vi "Pfeiffer-RVC300.ProcCases.vi"(0 "i ref in":refnum<vi>, 1 "selector":string, 2 "Data":T1, 3 "call cluster":T2={"Object"="", "Selector"="", "CallType"=enum."synchronous", "Async Object"="", "Async Selector"="", "Data Descriptor"="", "Data"=[], "Error #"=0, "Expire"=0}, 5 "error in (no error)":errorcluster) -> (14 "i ref out":refnum<vi>, 17 "answer cluster":T2={"Object"="", "Selector"="", "CallType"=enum."synchronous", "Async Object"="", "Async Selector"="", "Data Descriptor"="", "Data"=[], "Error #"=0, "Expire"=0}, 19 "error out":errorcluster)   [LabVIEW 2014, in "Pfeiffer-RVC300.lvlib"]
doc: "This method is called by a process from within the default case in the event loop. The methods of a class that are linked to events will be called from THIS method. Add your code here."
uses:
  Pfeiffer-RVC300.lvlib
  CS_Core/CSSystem/CoreLib/CoreLib.lvlib
  CS_Core/BaseProcess/BaseProcess.lvlib
  CS_Core/CSApplicationBaseClasses/DeviceBase/DeviceBase.lvlib
  CS_Core/CSSystem/CoreLib/CoreLib.string 2 byte array.vi
  CS_Core/CSSystem/CoreLib/CoreLib.byte array 2 double.vi
  CS_Core/CSSystem/CoreLib/CoreLib.double 2 byte array.vi
  CS_Core/CSSystem/CoreLib/CoreLib.byte array 2 short.vi
  CS_Core/CSSystem/CoreLib/CoreLib.int 2 byte array.vi
  CS_Core/CSSystem/CoreLib/CoreLib.byte array 2 int.vi
  CS_Core/CSSystem/CoreDefs/CoreDefs.call_type.ctl
  CS_Core/CSSystem/CoreDefs/CoreDefs.rawDataType.ctl
  CS_Core/BaseProcess/BaseProcess.descriptor string definition.ctl
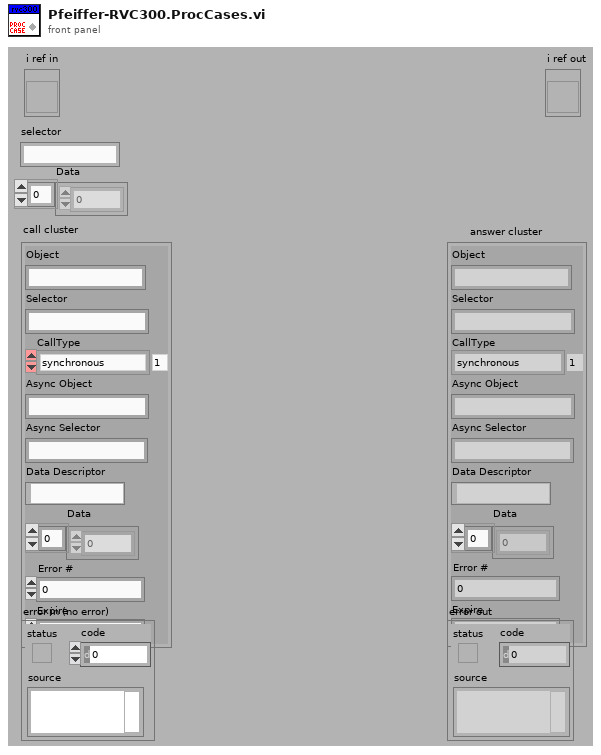
[diagram p1: front panel]
types:
  T1 = typedef "CoreDefs.rawDataType.ctl" = i8[]
  T2 = typedef "CoreDefs.call_type.ctl" = cluster{"Object":string, "Selector":string, "CallType":enum16{"simple", "synchronous", "asynchronous"}, "Async Object":string, "Async Selector":string, "Data Descriptor":T3, "Data":T1, "Error #":i32, "Expire":u32}
  T3 = typedef "BaseProcess.lvlib/BaseProcess.descriptor string definition.ctl" = string
  T4 = typedef "Pfeiffer-RVC300.lvlib/Pfeiffer-RVC300.regulation mode.ctl" = enum16{"unknown", "Pressure", "Flow", "Wait"}
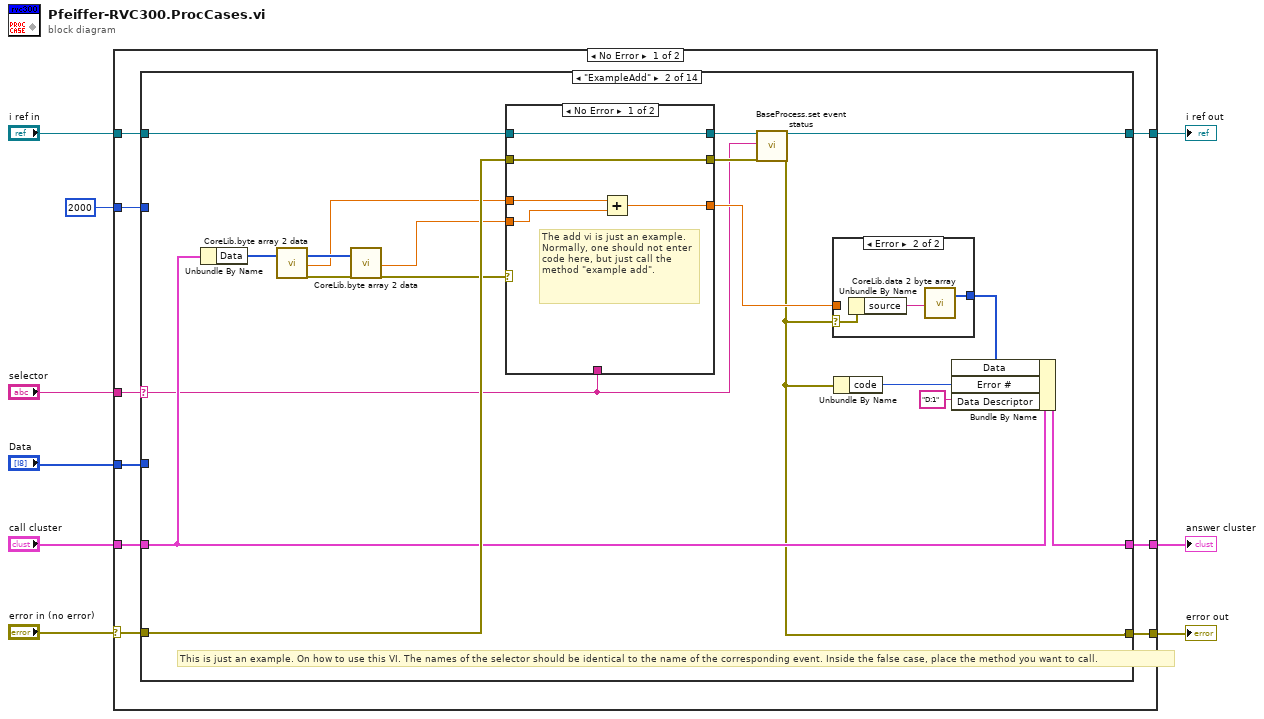
[diagram p0: block diagram]
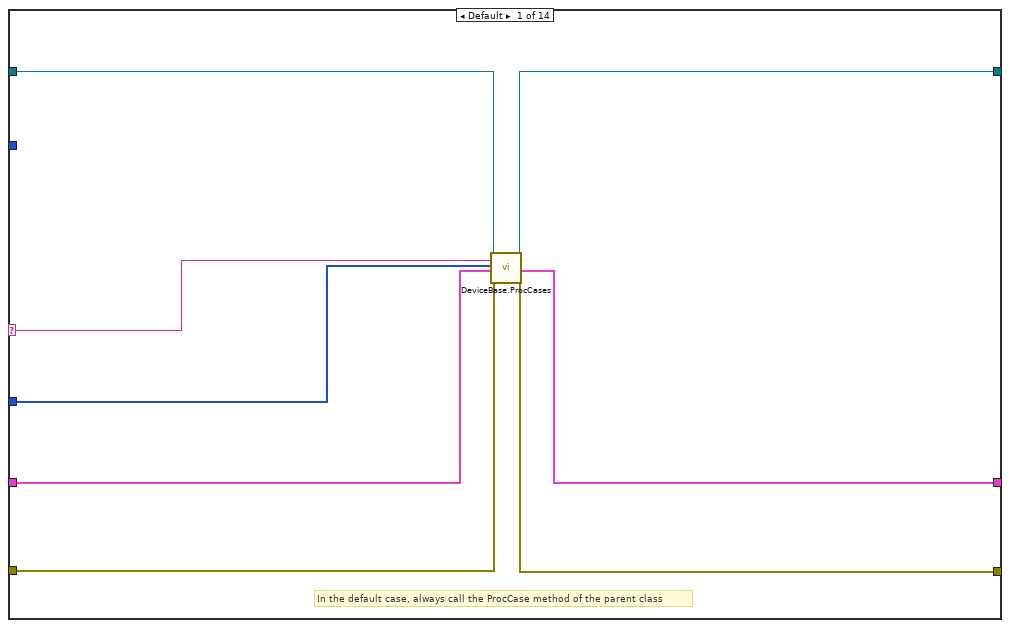
[diagram p2: hidden frame]
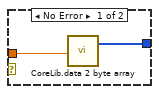
[diagram p3: hidden frame]
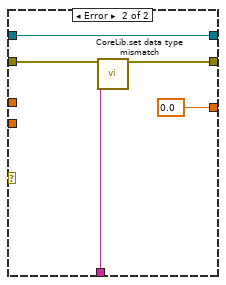
[diagram p4: hidden frame]
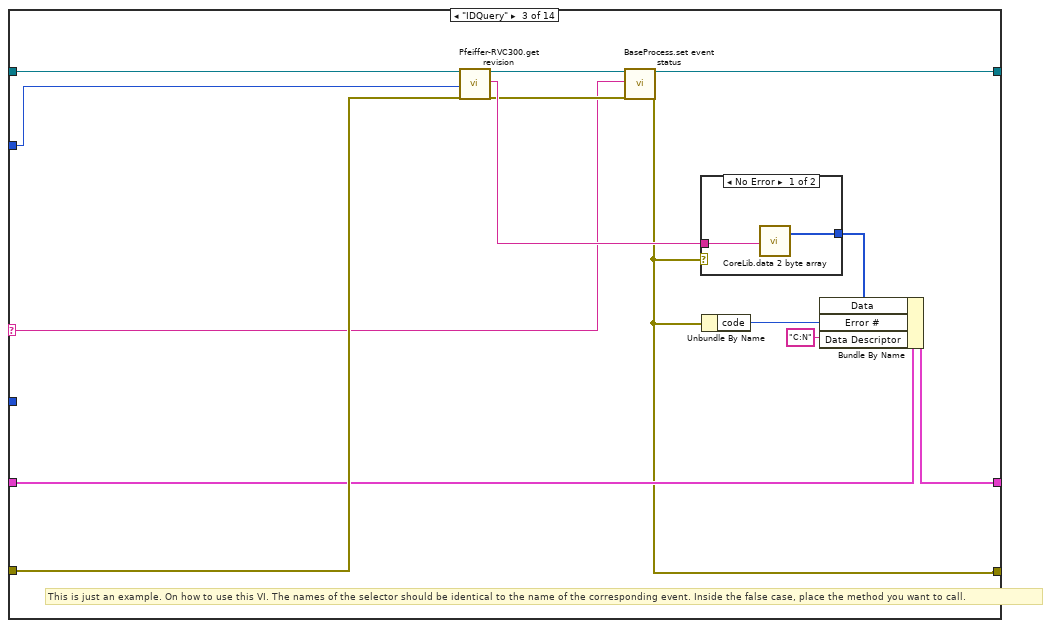
[diagram p5: hidden frame]
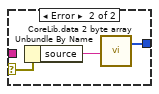
[diagram p6: hidden frame]
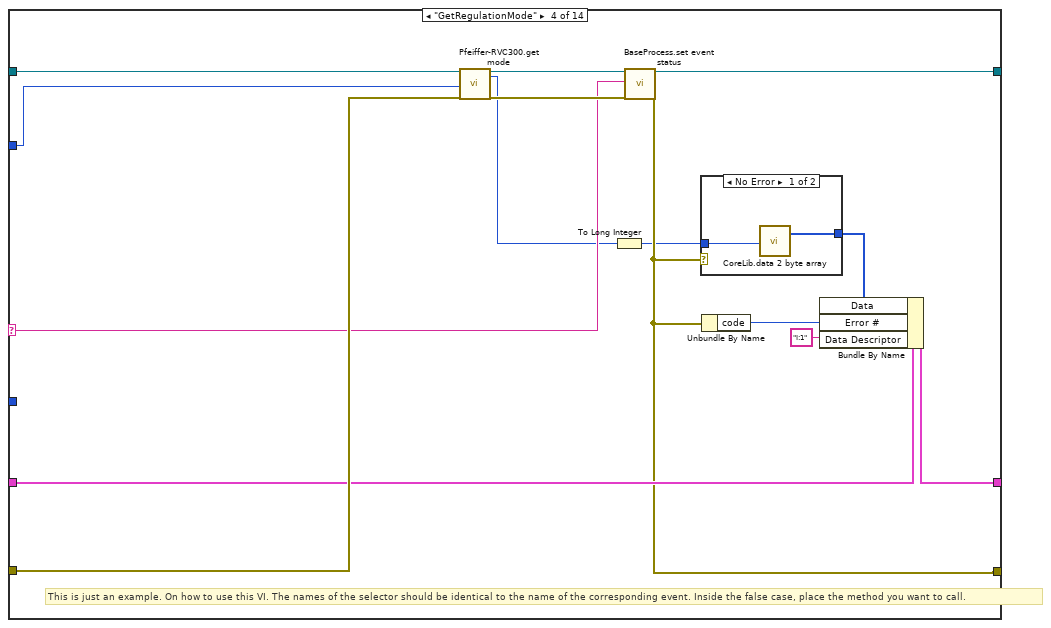
[diagram p7: hidden frame]
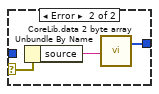
[diagram p8: hidden frame]
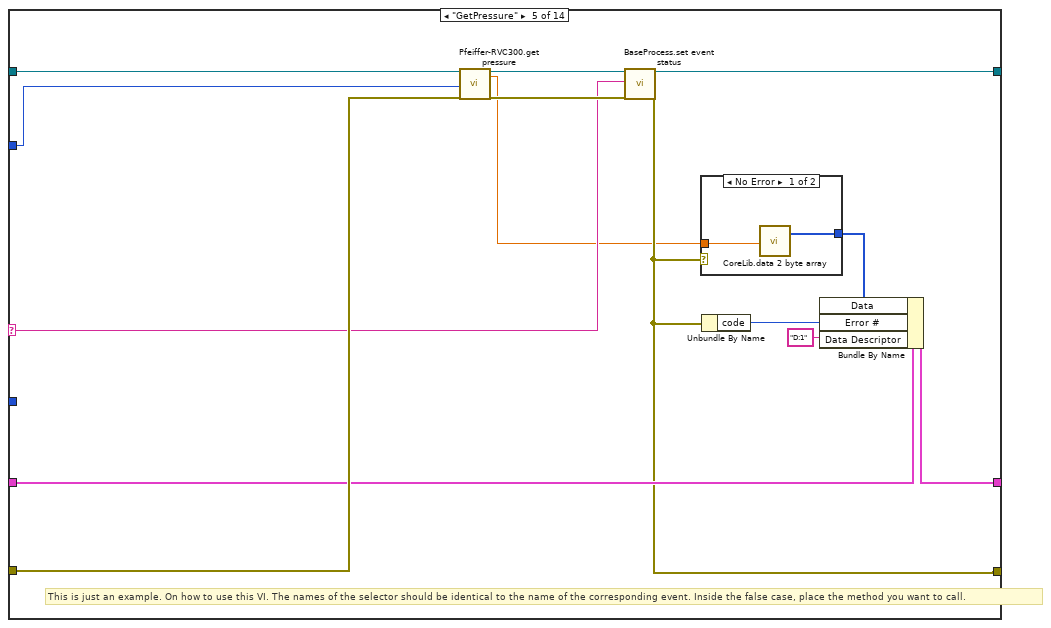
[diagram p9: hidden frame]
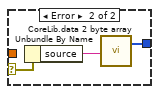
[diagram p10: hidden frame]
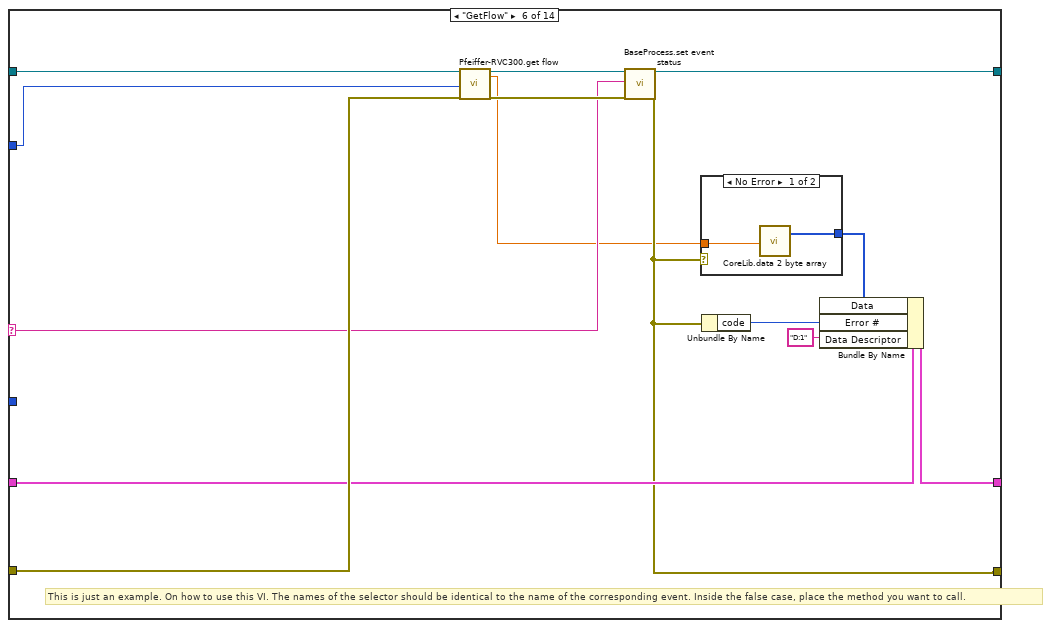
[diagram p11: hidden frame]
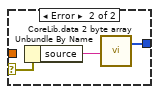
[diagram p12: hidden frame]
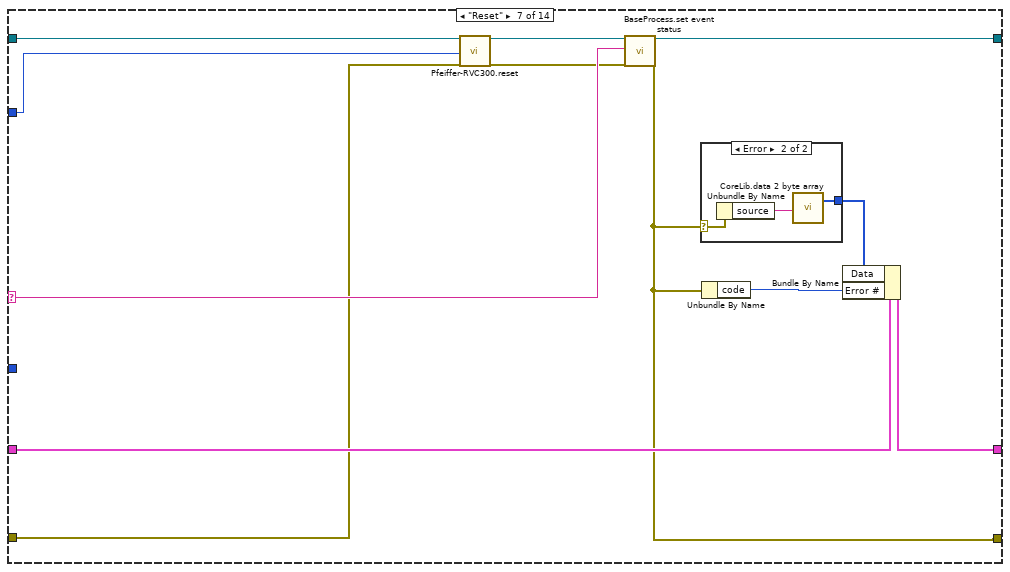
[diagram p13: hidden frame]
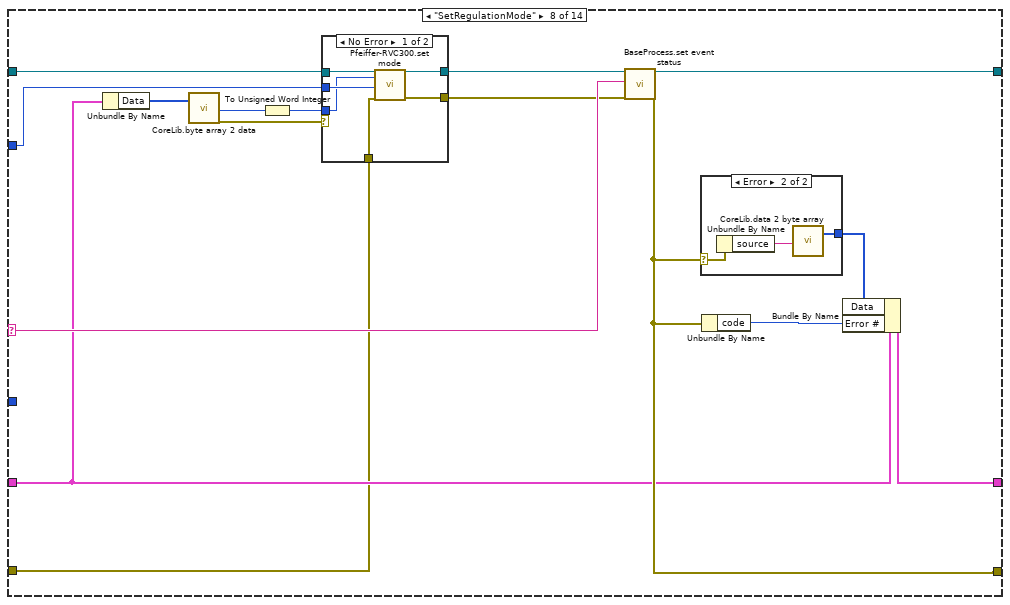
[diagram p15: hidden frame]
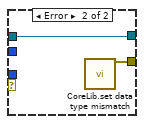
[diagram p16: hidden frame]
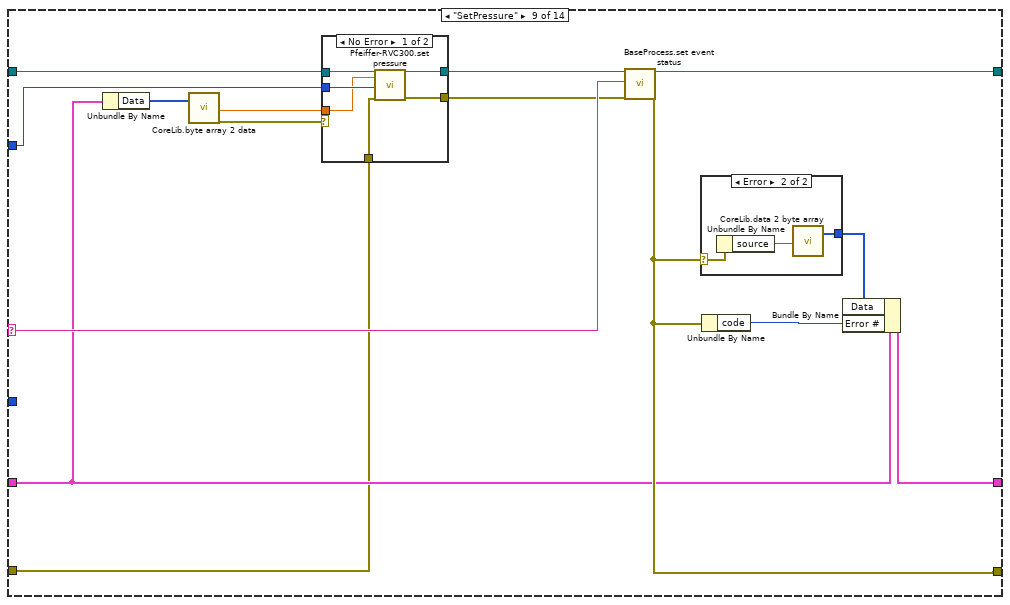
[diagram p18: hidden frame]
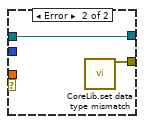
[diagram p19: hidden frame]
diagram:
  n1 = case shown="No Error" "error in (no error)" {
    selector: "error in (no error)" -> [w11 w314]
    tunnel: "selector" -> [w18 _]
    tunnel: [w17 w315] -> w8
    tunnel: "Data" -> [w16 _]
    tunnel: "call cluster" -> [w15 w315]
    tunnel: "i ref in" -> [w14 w316]
    tunnel: [w13 w316] -> w4
    tunnel: [w12 w314] -> w3
    tunnel: 2000 -> [w10 _]
    frame No Error {
      n2 = case shown="\"ExampleAdd\"" w18 {
        selector: w18 -> [w21 w35 w64 w85 w104 w123 w144 w163 w188 w213 w235 w250 w268 w301]
        tunnel: w16 -> [w19 _ _ _ _ _ _ _ _ _ _ _ _ _]
        tunnel: w14 -> [w20 w45 w74 w94 w113 w132 w142 w158 w183 w208 w233 w248 w278 w310]
        tunnel: [w26 w34 w63 w84 w103 w122 w143 w162 w187 w212 w234 w249 w267 w300] -> w13
        tunnel: w15 -> [w22 w41 w70 w91 w110 w129 w148 w159 w184 w209 w239 w254 w274 w307]
        tunnel: [w23 w40 w69 w90 w109 w128 w147 w166 w191 w216 w238 w253 w273 w306] -> w17
        tunnel: w11 -> [w25 w44 w73 w93 w112 w131 w139 w156 w181 w206 w230 w245 w277 w309]
        tunnel: [w24 w36 w65 w86 w105 w124 w145 w164 w189 w214 w236 w251 w269 w302] -> w12
        tunnel: w10 -> [_ _ w61 w82 w101 w120 w138 w154 w180 w205 w229 w244 w259 w299]
        frame Default {
          # "In the default case, always call the ProcCase method of the parent class"
          n3 = call "DeviceBase.ProcCases.vi"("i ref in"=w20, "selector"=w21, "Data"=w19, "call cluster"=w22, "error in (no error)"=w25) -> ("i ref out"=w26:refnum<vi>, "answer cluster"=w23:T2, "error out"=w24:errorcluster)  [unwired: 12 in]
        }
        frame "ExampleAdd" {
          # "This is just an example. On how to use this VI. The names of the selector should be identical to the name of the corresponding event. Inside the false case, place the method you want to call."
          n4 = Unbundle By Name(w41) -> ("Data"=w32:T1)
          n5 = call-poly "CoreLib.byte array 2 data.vi"("byteArray"=w32) -> ("byteArray out"=w30:T1, "d64"=w28:dbl, "error out"=w31:errorcluster)  [unwired: 16 in]
          n6 = call-poly "CoreLib.byte array 2 data.vi"("byteArray"=w30, "error in (no error)"=w31) -> ("d64"=w27:dbl, "error out"=w29:errorcluster)  [unwired: 15 in, 1 out]
          n7 = case shown="No Error" w29 {
            tunnel: [w52 w60] -> w38
            tunnel: w45 -> [w52 w60]
            tunnel: w44 -> [w53 w59]
            tunnel: [w53 w58] -> w37
            tunnel: w27 -> [w55 _]
            tunnel: [w54 0.0] -> w43
            tunnel: w35 -> [_ w56]
            tunnel: w28 -> [w51 _]
            frame No Error {
              # "The add vi is just an example. Normally, one should not enter code here, but just call the method \"example add\"."
              n8 = Add(x=w51, y=w55) -> (x+y=w54:dbl)
            }
            frame Error {
              n9 = call "CoreLib.set data type mismatch.vi"("error in (no error)"=w59, "error source"=w56) -> ("error out"=w58:errorcluster)  [unwired: 17 in]
            }
          }
          n10 = call "BaseProcess.set event status.vi"("i ref in"=w38, "EventStatus"=w35, "error in (no error)"=w37) -> ("i ref out"=w34:refnum<vi>, "error out"=w36:errorcluster)  [unwired: 14 in, 1 out]
          n11 = case shown="Error" w36 {
            selector: w36 -> [_ w50]
            tunnel: [w46 w49] -> w39
            tunnel: w43 -> [w47 _]
            frame No Error {
              n12 = call-poly "CoreLib.data 2 byte array.vi"("f64"=w47) -> ("byteArray out"=w46:T1)  [unwired: 18 in]
            }
            frame Error {
              n13 = Unbundle By Name(w50) -> ("source"=w48:string)
              n14 = call-poly "CoreLib.data 2 byte array.vi"("string"=w48) -> ("byteArray out"=w49:T1)  [unwired: 18 in]
            }
          }
          n15 = Unbundle By Name(w36) -> ("code"=w42:i32)
          n16 = Bundle By Name(cluster=w41, "Data"=w39, "Error #"=w42, "Data Descriptor"="D:1") -> (w40:T2)
        }
        frame "IDQuery" {
          # "This is just an example. On how to use this VI. The names of the selector should be identical to the name of the corresponding event. Inside the false case, place the method you want to call."
          n17 = call "Pfeiffer-RVC300.get revision.vi"("i ref in"=w74, "ms timeout (10000)"=w61, "error in (no error)"=w73) -> ("i ref out"=w67:refnum<vi>, "revision"=w72:string, "error out"=w66:errorcluster)  [unwired: 13 in, 1 out]
          n18 = call "BaseProcess.set event status.vi"("i ref in"=w67, "EventStatus"=w64, "error in (no error)"=w66) -> ("i ref out"=w63:refnum<vi>, "error out"=w65:errorcluster)  [unwired: 14 in, 1 out]
          n19 = case shown="No Error" w65 {
            selector: w65 -> [_ w79]
            tunnel: [w76 w78] -> w68
            tunnel: w72 -> [w75 _]
            frame No Error {
              n20 = call-poly "CoreLib.data 2 byte array.vi"("string"=w75) -> ("byteArray out"=w76:T1)  [unwired: 18 in]
            }
            frame Error {
              n21 = Unbundle By Name(w79) -> ("source"=w77:string)
              n22 = call-poly "CoreLib.data 2 byte array.vi"("string"=w77) -> ("byteArray out"=w78:T1)  [unwired: 18 in]
            }
          }
          n23 = Unbundle By Name(w65) -> ("code"=w71:i32)
          n24 = Bundle By Name(cluster=w70, "Data"=w68, "Error #"=w71, "Data Descriptor"="C:N") -> (w69:T2)
        }
        frame "GetRegulationMode" {
          # "This is just an example. On how to use this VI. The names of the selector should be identical to the name of the corresponding event. Inside the false case, place the method you want to call."
          n25 = call "Pfeiffer-RVC300.get mode.vi"("i ref in"=w94, "ms timeout (10000)"=w82, "error in (no error)"=w93) -> ("i ref out"=w88:refnum<vi>, "regulationMode"=w81:T4, "error out"=w87:errorcluster)  [unwired: 13 in, 1 out]
          n26 = To Long Integer(number=w81) -> (32bit integer=w80:i32)
          n27 = call "BaseProcess.set event status.vi"("i ref in"=w88, "EventStatus"=w85, "error in (no error)"=w87) -> ("i ref out"=w84:refnum<vi>, "error out"=w86:errorcluster)  [unwired: 14 in, 1 out]
          n28 = case shown="No Error" w86 {
            selector: w86 -> [_ w99]
            tunnel: [w96 w98] -> w89
            tunnel: w80 -> [w95 _]
            frame No Error {
              n29 = call-poly "CoreLib.data 2 byte array.vi"("i32"=w95) -> ("byteArray out"=w96:T1)  [unwired: 18 in]
            }
            frame Error {
              n30 = Unbundle By Name(w99) -> ("source"=w97:string)
              n31 = call-poly "CoreLib.data 2 byte array.vi"("string"=w97) -> ("byteArray out"=w98:T1)  [unwired: 18 in]
            }
          }
          n32 = Unbundle By Name(w86) -> ("code"=w92:i32)
          n33 = Bundle By Name(cluster=w91, "Data"=w89, "Error #"=w92, "Data Descriptor"="I:1") -> (w90:T2)
        }
        frame "GetPressure" {
          # "This is just an example. On how to use this VI. The names of the selector should be identical to the name of the corresponding event. Inside the false case, place the method you want to call."
          n34 = call "Pfeiffer-RVC300.get pressure.vi"("i ref in"=w113, "ms timeout (10000)"=w101, "error in (no error)"=w112) -> ("i ref out"=w107:refnum<vi>, "pressure"=w100:dbl, "error out"=w106:errorcluster)  [unwired: 13 in, 1 out]
          n35 = call "BaseProcess.set event status.vi"("i ref in"=w107, "EventStatus"=w104, "error in (no error)"=w106) -> ("i ref out"=w103:refnum<vi>, "error out"=w105:errorcluster)  [unwired: 14 in, 1 out]
          n36 = case shown="No Error" w105 {
            selector: w105 -> [_ w118]
            tunnel: [w115 w117] -> w108
            tunnel: w100 -> [w114 _]
            frame No Error {
              n37 = call-poly "CoreLib.data 2 byte array.vi"("f64"=w114) -> ("byteArray out"=w115:T1)  [unwired: 18 in]
            }
            frame Error {
              n38 = Unbundle By Name(w118) -> ("source"=w116:string)
              n39 = call-poly "CoreLib.data 2 byte array.vi"("string"=w116) -> ("byteArray out"=w117:T1)  [unwired: 18 in]
            }
          }
          n40 = Unbundle By Name(w105) -> ("code"=w111:i32)
          n41 = Bundle By Name(cluster=w110, "Data"=w108, "Error #"=w111, "Data Descriptor"="D:1") -> (w109:T2)
        }
        frame "GetFlow" {
          # "This is just an example. On how to use this VI. The names of the selector should be identical to the name of the corresponding event. Inside the false case, place the method you want to call."
          n42 = call "Pfeiffer-RVC300.get flow.vi"("i ref in"=w132, "ms timeout (10000)"=w120, "error in (no error)"=w131) -> ("i ref out"=w126:refnum<vi>, "flow"=w119:dbl, "error out"=w125:errorcluster)  [unwired: 13 in, 1 out]
          n43 = call "BaseProcess.set event status.vi"("i ref in"=w126, "EventStatus"=w123, "error in (no error)"=w125) -> ("i ref out"=w122:refnum<vi>, "error out"=w124:errorcluster)  [unwired: 14 in, 1 out]
          n44 = case shown="No Error" w124 {
            selector: w124 -> [_ w137]
            tunnel: [w134 w136] -> w127
            tunnel: w119 -> [w133 _]
            frame No Error {
              n45 = call-poly "CoreLib.data 2 byte array.vi"("f64"=w133) -> ("byteArray out"=w134:T1)  [unwired: 18 in]
            }
            frame Error {
              n46 = Unbundle By Name(w137) -> ("source"=w135:string)
              n47 = call-poly "CoreLib.data 2 byte array.vi"("string"=w135) -> ("byteArray out"=w136:T1)  [unwired: 18 in]
            }
          }
          n48 = Unbundle By Name(w124) -> ("code"=w130:i32)
          n49 = Bundle By Name(cluster=w129, "Data"=w127, "Error #"=w130, "Data Descriptor"="D:1") -> (w128:T2)
        }
        frame "Reset" {
          n50 = call "Pfeiffer-RVC300.reset.vi"("i ref in"=w142, "ms timeout (10000)"=w138, "error in (no error)"=w139) -> ("i ref out"=w141:refnum<vi>, "error out"=w140:errorcluster)  [unwired: 15 in]
          n51 = call "BaseProcess.set event status.vi"("i ref in"=w141, "EventStatus"=w144, "error in (no error)"=w140) -> ("i ref out"=w143:refnum<vi>, "error out"=w145:errorcluster)  [unwired: 14 in, 1 out]
          n52 = case shown="Error" w145 {
            selector: w145 -> [_ w152]
            tunnel: [_ w151] -> w146
            frame No Error {
            }
            frame Error {
              n53 = Unbundle By Name(w152) -> ("source"=w150:string)
              n54 = call-poly "CoreLib.data 2 byte array.vi"("string"=w150) -> ("byteArray out"=w151:T1)  [unwired: 18 in]
            }
          }
          n55 = Unbundle By Name(w145) -> ("code"=w149:i32)
          n56 = Bundle By Name(cluster=w148, "Data"=w146, "Error #"=w149) -> (w147:T2)
        }
        frame "SetRegulationMode" {
          n57 = Unbundle By Name(w159) -> ("Data"=w161:T1)
          n58 = call-poly "CoreLib.byte array 2 data.vi"("byteArray"=w161) -> ("i32"=w153:i32, "error out"=w160:errorcluster)  [unwired: 16 in, 1 out]
          n59 = To Unsigned Word Integer(number=w153) -> (unsigned 16bit integer=w155:u16)
          n60 = case shown="No Error" w160 {
            tunnel: w158 -> [w173 w175]
            tunnel: [w172 w175] -> _
            tunnel: [w171 w174] -> w157
            tunnel: w156 -> [w170 _]
            tunnel: w155 -> [w168 _]
            tunnel: w154 -> [w169 _]
            frame No Error {
              n61 = call "Pfeiffer-RVC300.set mode.vi"("i ref in"=w173, "regulationMode"=w168, "ms timeout (10000)"=w169, "error in (no error)"=w170) -> ("i ref out"=w172:refnum<vi>, "error out"=w171:errorcluster)  [unwired: 13 in, 1 out]
            }
            frame Error {
              n62 = call "CoreLib.set data type mismatch.vi"() -> ("error out"=w174:errorcluster)  [unwired: 19 in]
            }
          }
          n63 = call "BaseProcess.set event status.vi"("i ref in"=w158, "EventStatus"=w163, "error in (no error)"=w157) -> ("i ref out"=w162:refnum<vi>, "error out"=w164:errorcluster)  [unwired: 14 in, 1 out]
          n64 = case shown="Error" w164 {
            selector: w164 -> [_ w178]
            tunnel: [_ w177] -> w165
            frame No Error {
            }
            frame Error {
              n65 = Unbundle By Name(w178) -> ("source"=w176:string)
              n66 = call-poly "CoreLib.data 2 byte array.vi"("string"=w176) -> ("byteArray out"=w177:T1)  [unwired: 18 in]
            }
          }
          n67 = Unbundle By Name(w164) -> ("code"=w167:i32)
          n68 = Bundle By Name(cluster=w159, "Data"=w165, "Error #"=w167) -> (w166:T2)
        }
        frame "SetPressure" {
          n69 = Unbundle By Name(w184) -> ("Data"=w186:T1)
          n70 = call-poly "CoreLib.byte array 2 data.vi"("byteArray"=w186) -> ("d64"=w179:dbl, "error out"=w185:errorcluster)  [unwired: 16 in, 1 out]
          n71 = case shown="No Error" w185 {
            tunnel: w183 -> [w198 w200]
            tunnel: [w197 w200] -> _
            tunnel: [w196 w199] -> w182
            tunnel: w181 -> [w195 _]
            tunnel: w180 -> [w194 _]
            tunnel: w179 -> [w193 _]
            frame No Error {
              n72 = call "Pfeiffer-RVC300.set pressure.vi"("i ref in"=w198, "pressure"=w193, "ms timeout (10000)"=w194, "error in (no error)"=w195) -> ("i ref out"=w197:refnum<vi>, "error out"=w196:errorcluster)  [unwired: 13 in, 1 out]
            }
            frame Error {
              n73 = call "CoreLib.set data type mismatch.vi"() -> ("error out"=w199:errorcluster)  [unwired: 19 in]
            }
          }
          n74 = call "BaseProcess.set event status.vi"("i ref in"=w183, "EventStatus"=w188, "error in (no error)"=w182) -> ("i ref out"=w187:refnum<vi>, "error out"=w189:errorcluster)  [unwired: 14 in, 1 out]
          n75 = case shown="Error" w189 {
            selector: w189 -> [_ w203]
            tunnel: [_ w202] -> w190
            frame No Error {
            }
            frame Error {
              n76 = Unbundle By Name(w203) -> ("source"=w201:string)
              n77 = call-poly "CoreLib.data 2 byte array.vi"("string"=w201) -> ("byteArray out"=w202:T1)  [unwired: 18 in]
            }
          }
          n78 = Unbundle By Name(w189) -> ("code"=w192:i32)
          n79 = Bundle By Name(cluster=w184, "Data"=w190, "Error #"=w192) -> (w191:T2)
        }
        frame "SetFlow" {
          n80 = Unbundle By Name(w209) -> ("Data"=w211:T1)
          n81 = call-poly "CoreLib.byte array 2 data.vi"("byteArray"=w211) -> ("d64"=w204:dbl, "error out"=w210:errorcluster)  [unwired: 16 in, 1 out]
          n82 = case shown="No Error" w210 {
            tunnel: w208 -> [w223 w225]
            tunnel: [w222 w225] -> _
            tunnel: [w221 w224] -> w207
            tunnel: w206 -> [w220 _]
            tunnel: w205 -> [w219 _]
            tunnel: w204 -> [w218 _]
            frame No Error {
              n83 = call "Pfeiffer-RVC300.set flow.vi"("i ref in"=w223, "flow"=w218, "ms timeout (10000)"=w219, "error in (no error)"=w220) -> ("i ref out"=w222:refnum<vi>, "error out"=w221:errorcluster)  [unwired: 13 in, 1 out]
            }
            frame Error {
              n84 = call "CoreLib.set data type mismatch.vi"() -> ("error out"=w224:errorcluster)  [unwired: 19 in]
            }
          }
          n85 = call "BaseProcess.set event status.vi"("i ref in"=w208, "EventStatus"=w213, "error in (no error)"=w207) -> ("i ref out"=w212:refnum<vi>, "error out"=w214:errorcluster)  [unwired: 14 in, 1 out]
          n86 = case shown="Error" w214 {
            selector: w214 -> [_ w228]
            tunnel: [_ w227] -> w215
            frame No Error {
            }
            frame Error {
              n87 = Unbundle By Name(w228) -> ("source"=w226:string)
              n88 = call-poly "CoreLib.data 2 byte array.vi"("string"=w226) -> ("byteArray out"=w227:T1)  [unwired: 18 in]
            }
          }
          n89 = Unbundle By Name(w214) -> ("code"=w217:i32)
          n90 = Bundle By Name(cluster=w209, "Data"=w215, "Error #"=w217) -> (w216:T2)
        }
        frame "OpenValve" {
          n91 = call "Pfeiffer-RVC300.open valve.vi"("i ref in"=w233, "ms timeout (10000)"=w229, "error in (no error)"=w230) -> ("i ref out"=w232:refnum<vi>, "error out"=w231:errorcluster)  [unwired: 14 in, 1 out]
          n92 = call "BaseProcess.set event status.vi"("i ref in"=w232, "EventStatus"=w235, "error in (no error)"=w231) -> ("i ref out"=w234:refnum<vi>, "error out"=w236:errorcluster)  [unwired: 14 in, 1 out]
          n93 = case shown="Error" w236 {
            selector: w236 -> [_ w243]
            tunnel: [_ w242] -> w237
            frame No Error {
            }
            frame Error {
              n94 = Unbundle By Name(w243) -> ("source"=w241:string)
              n95 = call-poly "CoreLib.data 2 byte array.vi"("string"=w241) -> ("byteArray out"=w242:T1)  [unwired: 18 in]
            }
          }
          n96 = Unbundle By Name(w236) -> ("code"=w240:i32)
          n97 = Bundle By Name(cluster=w239, "Data"=w237, "Error #"=w240) -> (w238:T2)
        }
        frame "CloseValve" {
          n98 = call "Pfeiffer-RVC300.close valve.vi"("i ref in"=w248, "ms timeout (10000)"=w244, "error in (no error)"=w245) -> ("i ref out"=w247:refnum<vi>, "error out"=w246:errorcluster)  [unwired: 14 in, 1 out]
          n99 = call "BaseProcess.set event status.vi"("i ref in"=w247, "EventStatus"=w250, "error in (no error)"=w246) -> ("i ref out"=w249:refnum<vi>, "error out"=w251:errorcluster)  [unwired: 14 in, 1 out]
          n100 = case shown="Error" w251 {
            selector: w251 -> [_ w258]
            tunnel: [_ w257] -> w252
            frame No Error {
            }
            frame Error {
              n101 = Unbundle By Name(w258) -> ("source"=w256:string)
              n102 = call-poly "CoreLib.data 2 byte array.vi"("string"=w256) -> ("byteArray out"=w257:T1)  [unwired: 18 in]
            }
          }
          n103 = Unbundle By Name(w251) -> ("code"=w255:i32)
          n104 = Bundle By Name(cluster=w254, "Data"=w252, "Error #"=w255) -> (w253:T2)
        }
        frame "Initialize" {
          n105 = Unbundle By Name(w274) -> ("Data"=w265:T1)
          n106 = call-poly "CoreLib.byte array 2 data.vi"("byteArray"=w265) -> ("byteArray out"=w263:T1, "i16"=w261:i16, "error out"=w264:errorcluster)  [unwired: 16 in]
          n107 = call-poly "CoreLib.byte array 2 data.vi"("byteArray"=w263, "error in (no error)"=w264) -> ("i16"=w260:i16, "error out"=w262:errorcluster)  [unwired: 15 in, 1 out]
          n108 = case shown="No Error" w262 {
            tunnel: [w290 w298] -> w271
            tunnel: w278 -> [w293 w298]
            tunnel: w277 -> [w292 w297]
            tunnel: [w291 w296] -> w270
            tunnel: w260 -> [w288 _]
            tunnel: [w285 "N/A" ("deviceID")] -> w276
            tunnel: w268 -> [_ w295]
            tunnel: w261 -> [w289 _]
            tunnel: w259 -> [w284 _]
            frame No Error {
              n109 = Not Equal To 0?(x=w289) -> (x != 0?=w287:bool)
              n110 = Not Equal To 0?(x=w288) -> (x != 0?=w286:bool)
              n111 = call "Pfeiffer-RVC300.initialize interface.vi"("i ref in"=w293, "queryID"=w287, "resetDevice"=w286, "ms timeout (10000)"=w284, "error in (no error)"=w292) -> ("i ref out"=w290:refnum<vi>, "deviceID"=w285:string, "error out"=w291:errorcluster)  [unwired: 11 in, 1 out]
            }
            frame Error {
              n112 = call "CoreLib.set data type mismatch.vi"("error in (no error)"=w297, "error source"=w295) -> ("error out"=w296:errorcluster)  [unwired: 17 in]
            }
          }
          n113 = call "BaseProcess.set event status.vi"("i ref in"=w271, "EventStatus"=w268, "error in (no error)"=w270) -> ("i ref out"=w267:refnum<vi>, "error out"=w269:errorcluster)  [unwired: 14 in, 1 out]
          n114 = case shown="No Error" w269 {
            selector: w269 -> [_ w283]
            tunnel: [w279 w282] -> w272
            tunnel: w276 -> [w280 _]
            frame No Error {
              n115 = call-poly "CoreLib.data 2 byte array.vi"("string"=w280) -> ("byteArray out"=w279:T1)  [unwired: 18 in]
            }
            frame Error {
              n116 = Unbundle By Name(w283) -> ("source"=w281:string)
              n117 = call-poly "CoreLib.data 2 byte array.vi"("string"=w281) -> ("byteArray out"=w282:T1)  [unwired: 18 in]
            }
          }
          n118 = Unbundle By Name(w269) -> ("code"=w275:i32)
          n119 = Bundle By Name(cluster=w274, "Data"=w272, "Error #"=w275, "Data Descriptor"="C:N") -> (w273:T2)
        }
        frame "Close" {
          n120 = call "Pfeiffer-RVC300.close interface.vi"("i ref in"=w310, "ms timeout (10000)"=w299, "error in (no error)"=w309) -> ("i ref out"=w304:refnum<vi>, "error out"=w303:errorcluster)  [unwired: 14 in, 1 out]
          n121 = call "BaseProcess.set event status.vi"("i ref in"=w304, "EventStatus"=w301, "error in (no error)"=w303) -> ("i ref out"=w300:refnum<vi>, "error out"=w302:errorcluster)  [unwired: 14 in, 1 out]
          n122 = case shown="No Error" w302 {
            selector: w302 -> [_ w313]
            tunnel: [_ w312] -> w305
            frame No Error {
            }
            frame Error {
              n123 = Unbundle By Name(w313) -> ("source"=w311:string)
              n124 = call-poly "CoreLib.data 2 byte array.vi"("string"=w311) -> ("byteArray out"=w312:T1)  [unwired: 18 in]
            }
          }
          n125 = Unbundle By Name(w302) -> ("code"=w308:i32)
          n126 = Bundle By Name(cluster=w307, "Data"=w305, "Error #"=w308) -> (w306:T2)
        }
      }
    }
    frame Error {
    }
  }
  "answer cluster" <- w8
  "i ref out" <- w4
  "error out" <- w3
